vi "ConnectionStatus.vi"(8 "MCU_status":bool=TRUE, 9 "PSU_status":bool, 10 "Camera_status":bool, 11 "cDAQ_Therm_status":bool=TRUE) -> (0 "String":string, 3 "Status":bool)   [LabVIEW 2024]
panel:
  out "MCU":string="Micro Controller Unit"
  out "MCU":bool=TRUE
  out "TCam":string="Thermal Camera"
  out "PSU":string="Power Supply"
  out "cDAQ":string="cDAQ"
  out "PSU":bool
  in  "Connect":bool
  out "Cam":bool
  out "cDAQ Therm":bool=TRUE
  in  "OK":bool
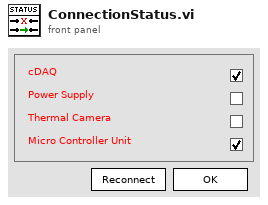
[diagram p1: front panel]
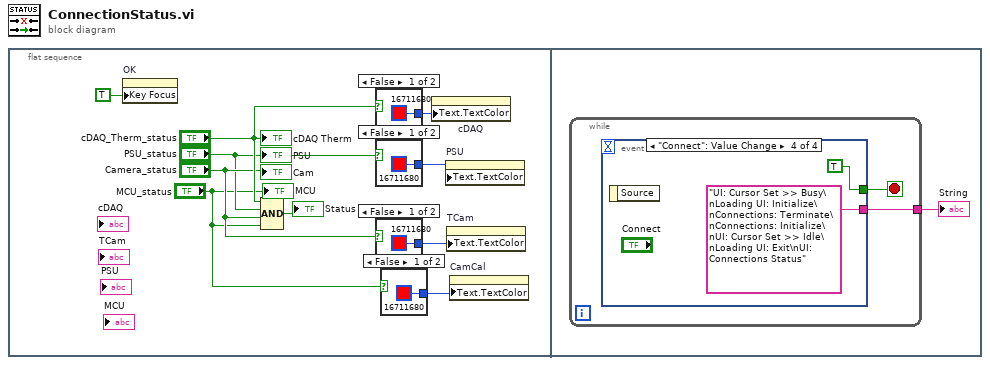
[diagram p0: block diagram]
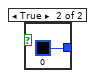
[diagram p2: hidden frame]
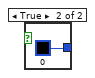
[diagram p3: hidden frame]
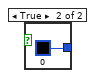
[diagram p4: hidden frame]
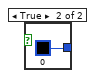
[diagram p5: hidden frame]
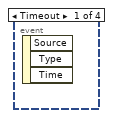
[diagram p6: hidden frame]
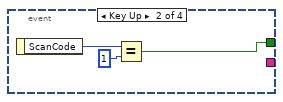
[diagram p7: hidden frame]
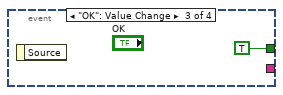
[diagram p8: hidden frame]
diagram:
  n1 = flat-sequence {
    frame #0 {
      n2 = property on="OK" class="Bool"("Key Focus"=TRUE) -> ()  [unwired: 2 in, 2 out]
      n3 = Compound Arithmetic op=AND("cDAQ_Therm_status", "PSU_status", "Camera_status", "MCU_status") -> (→"Status":bool)
      n4 = case shown="False" "cDAQ_Therm_status" {
        tunnel: [u32 16711680 ("Text.Text Colors:Text Color") u32 0 ("Text.Text Colors:Text Color")] -> w7
        frame False {
        }
        frame True {
        }
      }
      n5 = case shown="False" "PSU_status" {
        tunnel: [u32 16711680 ("Text.Text Colors:Text Color") u32 0 ("Text.Text Colors:Text Color")] -> w4
        frame False {
        }
        frame True {
        }
      }
      n6 = case shown="False" "Camera_status" {
        tunnel: [u32 16711680 ("Text.Text Colors:Text Color") u32 0 ("Text.Text Colors:Text Color")] -> w6
        frame False {
        }
        frame True {
        }
      }
      n7 = case shown="False" "MCU_status" {
        tunnel: [u32 16711680 ("Text.Text Colors:Text Color") u32 0 ("Text.Text Colors:Text Color")] -> w1
        frame False {
        }
        frame True {
        }
      }
      n8 = property on="cDAQ" class="Str"("Text.TextColor"=w7) -> ()  [unwired: 2 in, 2 out]
      n9 = property on="PSU" class="Str"("Text.TextColor"=w4) -> ()  [unwired: 2 in, 2 out]
      n10 = property on="TCam" class="Str"("Text.TextColor"=w6) -> ()  [unwired: 2 in, 2 out]
      n11 = property on="CamCal" class="Str"("Text.TextColor"=w1) -> ()  [unwired: 2 in, 2 out]
      "cDAQ Therm" <- "cDAQ_Therm_status"
      "Cam" <- "Camera_status"
      "PSU" <- "PSU_status"
      "MCU" <- "MCU_status"
    }
    frame #1 {
      n12 = while {
        tunnel: [w20] -> w19
        stop <- w21 stop-if-true
        n13 = event shown="[3] \"Connect\": Value Change" {
          selector: _ -> [_ _ _ _]
          dyn-events: _ -> [_ _ _ _]
          timeout: _ -> [_ _ _ _]
          tunnel: [_ w22 TRUE TRUE] -> w21
          tunnel: [_ _ _ "UI: Cursor Set >> Busy\nLoading UI: Initialize\nConnections: Terminate\nConnections: Initialize\nUI: Cursor Set >> Idle\nLoading UI: Exit\nUI: Connections Status"] -> w20
          event Timeout {
            n14 = event-data() -> ()  [unwired: 1 in, 3 out]
          }
          event Key Up {
            n15 = event-data() -> ("ScanCode"=w24:i16)  [unwired: 1 in]
            n16 = Equal?(x=w24, y=i16 1) -> (x = y?=w22:bool)
          }
          event "OK": Value Change {
            n17 = event-data() -> ()  [unwired: 1 in, 1 out]
          }
          event "Connect": Value Change {
            n18 = event-data() -> ()  [unwired: 1 in, 1 out]
          }
        }
      }
      "String" <- w19
    }
  }
